vi "Parse Arguments.vi"(9 "Working Directory":path, 10 "Command Line Args":string[](array[string]), 11 "Parameters in":T1) -> (0 "error constant":errorcluster, 3 "Parameters out":T1)   [LabVIEW 2016]
uses:
  Typedefs/Command Line Arguments.ctl
  <vilib>/regexp/Match Regular Expression.xnode
  <vilib>/ErrorRing/Error Ring.xnode
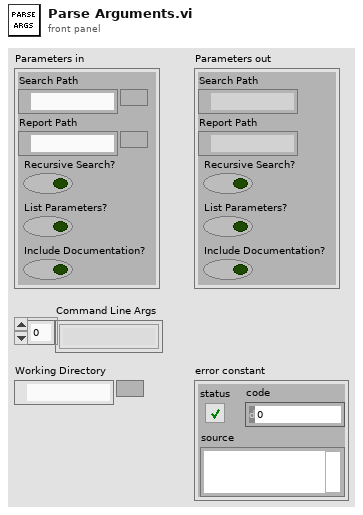
[diagram p1: front panel]
types:
  T1 = typedef "Command Line Arguments.ctl" = cluster{"Search Path":path, "Report Path":path, "Recursive Search?":bool, "List Parameters?":bool, "Include Documentation?":bool}
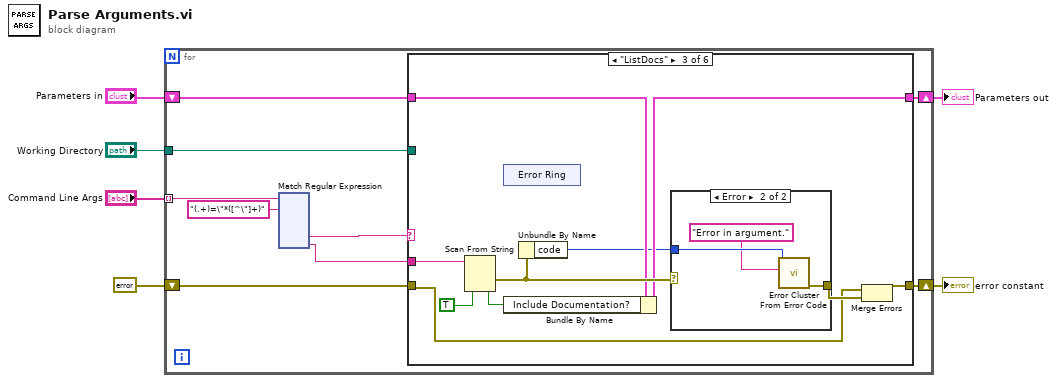
[diagram p0: block diagram]
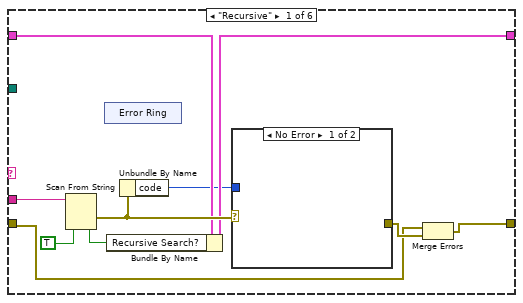
[diagram p2: hidden frame]
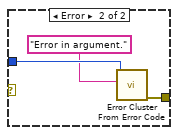
[diagram p3: hidden frame]
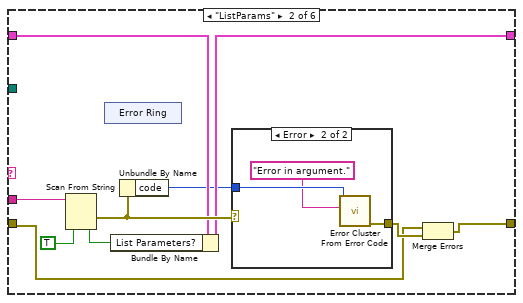
[diagram p4: hidden frame]
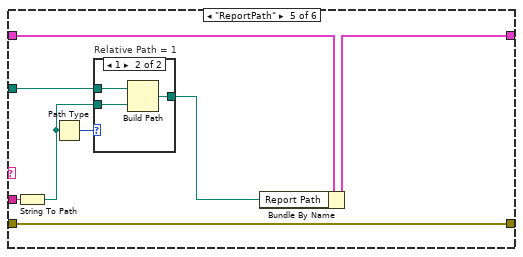
[diagram p8: hidden frame]
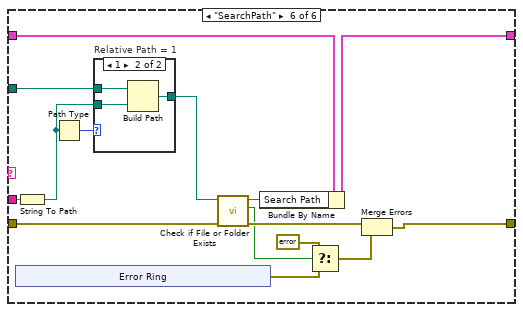
[diagram p10: hidden frame]
diagram:
  n1 = for {
    tunnel: "Command Line Args" -> [w10] mode=indexing
    shift-right: [w12] -> w3
    shift-left: "Parameters in" -> [w13]
    shift-right: [w14] -> w5
    shift-left: errorcluster {"status"=FALSE, "code"=0, "source"=""} ("error constant") -> [w15]
    tunnel: "Working Directory" -> [w7]
    n2 = xnode "Match Regular Expression"("input string"=w10, "regular expression"="(.+)=\"*([^\"]+)") -> ("submatch 1"=w9:string, "submatch 2"=w8:string)  [unwired: 4 in, 5 out]
    n3 = case shown="\"ListDocs\"" w9 {
      tunnel: w8 -> [w137 w151 w165 _ w182 w195]
      tunnel: w13 -> [w138 w152 w166 w175 w184 w197]
      tunnel: [w135 w149 w163 w175 w183 w196] -> w12
      tunnel: w15 -> [w139 w153 w167 w176 w177 w203]
      tunnel: [w140 w154 w168 w176 w177 w201] -> w14
      tunnel: w7 -> [_ _ _ _ w180 w191]
      frame "Recursive" {
        n4 = Scan From String(input string=w137, default 1=TRUE) -> (error out=w141:errorcluster, output 1=w134:bool)  [unwired: 3 in, 2 out]
        n5 = xnode "Error Ring"() -> ()  [unwired: 1 out]
        n6 = Bundle By Name(cluster=w138, "Recursive Search?"=w134) -> (w135:T1)
        n7 = Unbundle By Name(w141) -> ("code"=w133:i32)
        n8 = case shown="No Error" w141 {
          tunnel: [_ w146] -> w142
          tunnel: w133 -> [_ w145]
          frame No Error {
          }
          frame Error {
            n9 = call <vilib>:"Error Cluster From Error Code.vi"("error message (\"\")"="Error in argument." ("error message (\"\")"), "error code (0)"=w145) -> ("error out"=w146:errorcluster)  [unwired: 7 in]
          }
        }
        n10 = Merge Errors(w139, w142) -> (w140:errorcluster)
      }
      frame "ListParams" {
        n11 = Scan From String(input string=w151, default 1=TRUE) -> (error out=w155:errorcluster, output 1=w148:bool)  [unwired: 3 in, 2 out]
        n12 = xnode "Error Ring"() -> ()  [unwired: 1 out]
        n13 = Bundle By Name(cluster=w152, "List Parameters?"=w148) -> (w149:T1)
        n14 = Unbundle By Name(w155) -> ("code"=w147:i32)
        n15 = case shown="Error" w155 {
          tunnel: [_ w160] -> w156
          tunnel: w147 -> [_ w159]
          frame No Error {
          }
          frame Error {
            n16 = call <vilib>:"Error Cluster From Error Code.vi"("error message (\"\")"="Error in argument." ("error message (\"\")"), "error code (0)"=w159) -> ("error out"=w160:errorcluster)  [unwired: 7 in]
          }
        }
        n17 = Merge Errors(w153, w156) -> (w154:errorcluster)
      }
      frame "ListDocs" {
        n18 = Scan From String(input string=w165, default 1=TRUE) -> (error out=w169:errorcluster, output 1=w162:bool)  [unwired: 3 in, 2 out]
        n19 = xnode "Error Ring"() -> ()  [unwired: 1 out]
        n20 = Bundle By Name(cluster=w166, "Include Documentation?"=w162) -> (w163:T1)
        n21 = Unbundle By Name(w169) -> ("code"=w161:i32)
        n22 = case shown="Error" w169 {
          tunnel: [_ w174] -> w170
          tunnel: w161 -> [_ w173]
          frame No Error {
          }
          frame Error {
            n23 = call <vilib>:"Error Cluster From Error Code.vi"("error message (\"\")"="Error in argument." ("error message (\"\")"), "error code (0)"=w173) -> ("error out"=w174:errorcluster)  [unwired: 7 in]
          }
        }
        n24 = Merge Errors(w167, w170) -> (w168:errorcluster)
      }
      frame Default {
      }
      frame "ReportPath" {
        n25 = String To Path(string=w182) -> (path=w179:path)
        n26 = Path Type(1:w179) -> (0:w181:i16)
        n27 = case "Relative Path = 1" shown="1" w181 {
          tunnel: w180 -> [_ w188]
          tunnel: w179 -> [w185 w187]
          tunnel: [w185 w186] -> w178
          frame Default {
          }
          frame 1 {
            n28 = Build Path(base path=w188, name or relative path=w187) -> (appended path=w186:path)
          }
        }
        n29 = Bundle By Name(cluster=w184, "Report Path"=w178) -> (w183:T1)
      }
      frame "SearchPath" {
        n30 = xnode "Error Ring"() -> ("error out"=w200:errorcluster)
        n31 = String To Path(string=w195) -> (path=w190:path)
        n32 = Path Type(1:w190) -> (0:w192:i16)
        n33 = case "Relative Path = 1" shown="1" w192 {
          tunnel: w191 -> [_ w207]
          tunnel: w190 -> [w204 w206]
          tunnel: [w204 w205] -> w189
          frame Default {
          }
          frame 1 {
            n34 = Build Path(base path=w207, name or relative path=w206) -> (appended path=w205:path)
          }
        }
        n35 = call <vilib>:"Check if File or Folder Exists.vi"("error in (no error)"=w203, "path"=w189) -> ("error out"=w202:errorcluster, "file or folder exists?"=w193:bool, "dup path"=w194:path)  [unwired: 7 in]
        n36 = Bundle By Name(cluster=w197, "Search Path"=w194) -> (w196:T1)
        n37 = Select(t=errorcluster {"status"=FALSE, "code"=0, "source"=""} ("error constant"), s=w193, f=w200) -> (s? t:f=w198:errorcluster)
        n38 = Merge Errors(w202, w198) -> (w201:errorcluster)
      }
    }
  }
  "Parameters out" <- w3
  "error constant" <- w5
